vi "Read Timestamp.vi"(8 "error in (no error)":errorcluster, 11 "Printf_Msg_General in":refnum<class "LV_Printf Msg.lvclass">) -> (0 "error out":errorcluster, 2 "Timestamp":timestamp, 3 "Printf_Msg_General out":refnum<class "LV_Printf Msg.lvclass">)   [LabVIEW 2013, in "SET_Printf.lvlib" / "LV_Printf Msg.lvclass"]
uses:
  LV_Printf Msg.lvclass
  LV_Printf Msg.lvclass/LV_Printf Msg.ctl
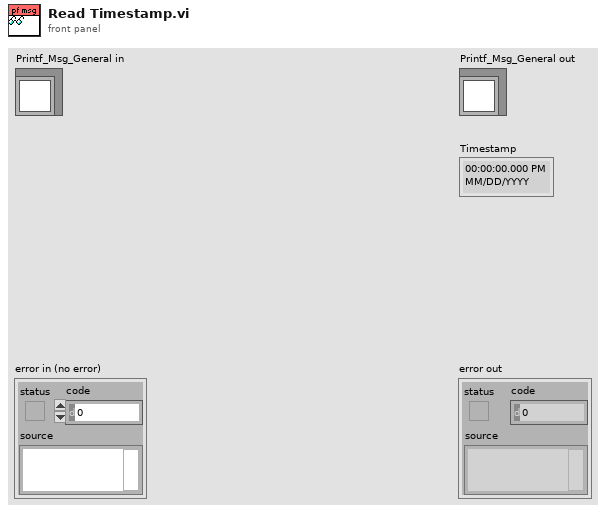
[diagram p1: front panel]
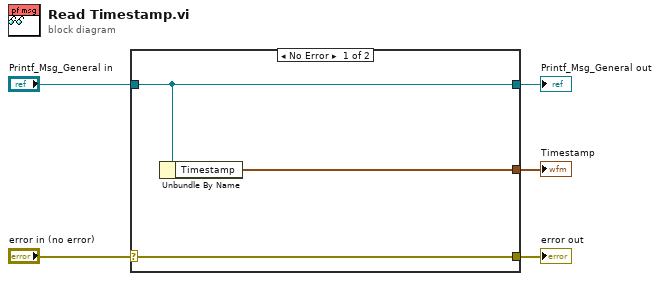
[diagram p0: block diagram]
diagram:
  n1 = case shown="No Error" "error in (no error)" {
    selector: "error in (no error)" -> [w8 w9]
    tunnel: [w8 w9] -> w4
    tunnel: [w7 w10] -> w2
    tunnel: "Printf_Msg_General in" -> [w7 w10]
    tunnel: [w6 _] -> w1
    frame No Error {
      n2 = Unbundle By Name(w7) -> ("Timestamp"=w6:timestamp)
    }
    frame Error {
    }
  }
  "error out" <- w4
  "Printf_Msg_General out" <- w2
  "Timestamp" <- w1
